vi "confirmSetpointApplied.vi"(8 "error in (no error)":errorcluster, 10 "model":refnum<class "Model.lvclass">, 11 "AwaitingSetpointAcknowledgmentState in":refnum<class "AwaitingSetpointAcknowledgmentState.lvclass">) -> (0 "error out":errorcluster, 2 "model 2":refnum<class "Model.lvclass">, 3 "AwaitingSetpointAcknowledgmentState out":refnum<class "AwaitingSetpointAcknowledgmentState.lvclass">)   [LabVIEW 2013, in "AwaitingSetpointAcknowledgmentState.lvclass"]
uses:
  AwaitingSetpointAcknowledgmentState.lvclass
  Model/Model/Model.lvclass
  Typedefs/StateSelector.ctl
  MovingToNewTemperatureState/MovingToNewTemperatureState.lvclass
  Typedefs/AITDTTypedefs.lvlib
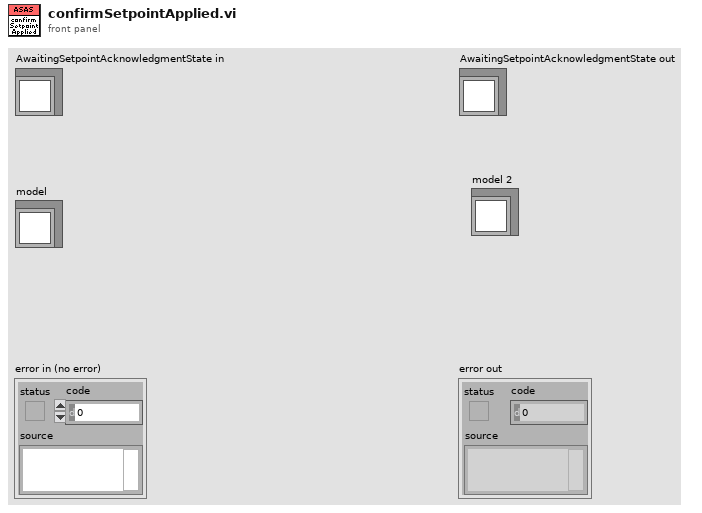
[diagram p1: front panel]
types:
  T1 = typedef "AITDTTypedefs.lvlib/StateSelector.ctl" = enum16{"AwaitingSetpointAcknowledgmentState", "EndingCycleState", "FaultState", "OffState", "PausingState", "RequestingNewSetpointState", "SamplingState", "SettlingState", "SoakingState", "StabilizingState", "StandbyState", "StoppedState", "TransitioningTemperatureState"}
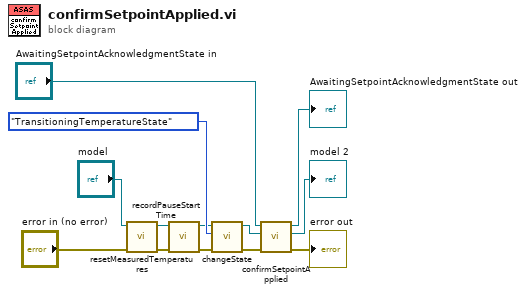
[diagram p0: block diagram]
diagram:
  n1 = call "resetMeasuredTemperatures.vi"("error in (no error)"="error in (no error)", "Model in"="model") -> ("error out"=w4:errorcluster, "Model out"=w2:refnum<class "Model.lvclass">)  [unwired: 8 in]
  n2 = call "recordPauseStartTime.vi"("error in (no error)"=w4, "Model in"=w2) -> ("error out"=w9:errorcluster, "Model out"=w8:refnum<class "Model.lvclass">)  [unwired: 8 in]
  n3 = call "changeState.vi"("error in (no error)"=w9, "State:"=StateSelector."TransitioningTemperatureState", "Model in"=w8) -> ("error out"=w5:errorcluster, "Model out"=w6:refnum<class "Model.lvclass">)  [unwired: 7 in]
  n4 = call-parent "confirmSetpointApplied.vi"("error in (no error)"=w5, "model"=w6, "State in"="AwaitingSetpointAcknowledgmentState in") -> ("error out"=→"error out":errorcluster, "model 2"=→"model 2":refnum<class "Model.lvclass">, "State out"=→"AwaitingSetpointAcknowledgmentState out":refnum<class "AwaitingSetpointAcknowledgmentState.lvclass">)  [unwired: 6 in]
